vi "Untitled 3.vi"() -> ()   [LabVIEW 2024]
panel:
  out "data":dbl
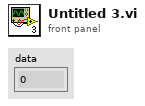
[diagram p1: front panel]
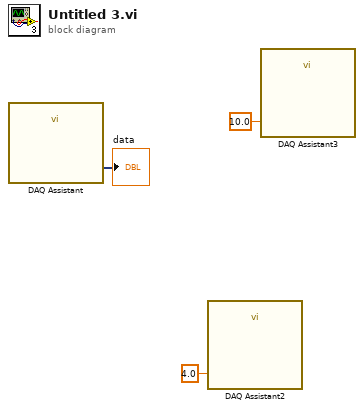
[diagram p0: block diagram]
diagram:
  n1 = call "DAQ Assistant"() -> ("data"=→"data":dynamicdata)  [unwired: 17 in, 2 out]
  n2 = call "DAQ Assistant2"("data"=4.0) -> ()  [unwired: 17 in, 2 out]
  n3 = call "DAQ Assistant3"("data"=10.0) -> ()  [unwired: 17 in, 2 out]
